vi "Main VI.vi"(8 "error in":errorcluster) -> (0 "error out":errorcluster)   [LabVIEW 2021]
doc: "Basic calculator built with LabVIEW"
uses:
  Controls/Queue Element.ctl
  Controls/Command Enum.ctl
  Controls/Storage Commands.ctl
  Controls/Storing Commands.ctl
  Controls/String Commands.ctl
  Controls/Operator String Control.ctl
  Controls/Operator Types.ctl
  Controls/String-Double Conversion Control.ctl
  Controls/Calculation Commands.ctl
panel:
  in  "Square":bool
  in  "Negate":bool
  in  "Clear All":bool
  in  "Clear Line":bool
  in  "Backspace":bool
  out "Secondary":string
  out "Primary":string
  in  "Square Root":bool
  in  "Reciprocal":bool
  in  "Equals":bool
  in  "Divide":bool
  in  "Multiply":bool
  in  "Subtract":bool
  in  "Add":bool
  in  "Decimal Point":bool
  in  "Button 0":bool
  in  "Button 9":bool
  in  "Button 8":bool
  in  "Button 7":bool
  in  "Button 6":bool
  in  "Button 5":bool
  in  "Button 4":bool
  in  "Button 3":bool
  in  "Button 2":bool
  in  "Button 1":bool
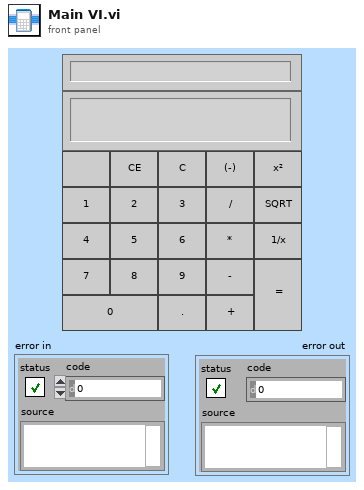
[diagram p1: front panel]
types:
  T1 = typedef "Queue Element.ctl" = cluster{"Command":T2, "Parameter":variant}
  T2 = typedef "Command Enum.ctl" = enum16{"Initialise", "Data Entry", "Decimal Point", "Operator", "Calculation", "Backspace", "Clear Line", "Clear All", "Close"}
  T3 = typedef "Operator String Control.ctl" = enum16{"GET", "Build", "Clear"}
  T4 = typedef "String Commands.ctl" = enum16{"GET Strings", "Set Secondary", "Build Primary", "Build Secondary", "Backspace", "Replace Operator", "Clear Primary", "Clear Secondary", "Clear ALL", "Decimal Point"}
  T5 = typedef "Storing Commands.ctl" = enum16{"Initialise", "GET", "SET"}
  T6 = typedef "Storage Commands.ctl" = enum16{"Initialise", "Build", "GET", "Reset"}
  T7 = typedef "Operator Types.ctl" = enum16{"Add", "Subtract", "Multiply", "Divide"}
  T8 = typedef "String-Double Conversion Control.ctl" = enum16{"String to DBL", "DBL to String"}
  T9 = typedef "Calculation Commands.ctl" = enum16{"Equals", "Square", "Square Root", "Reciprocal", "Negate"}
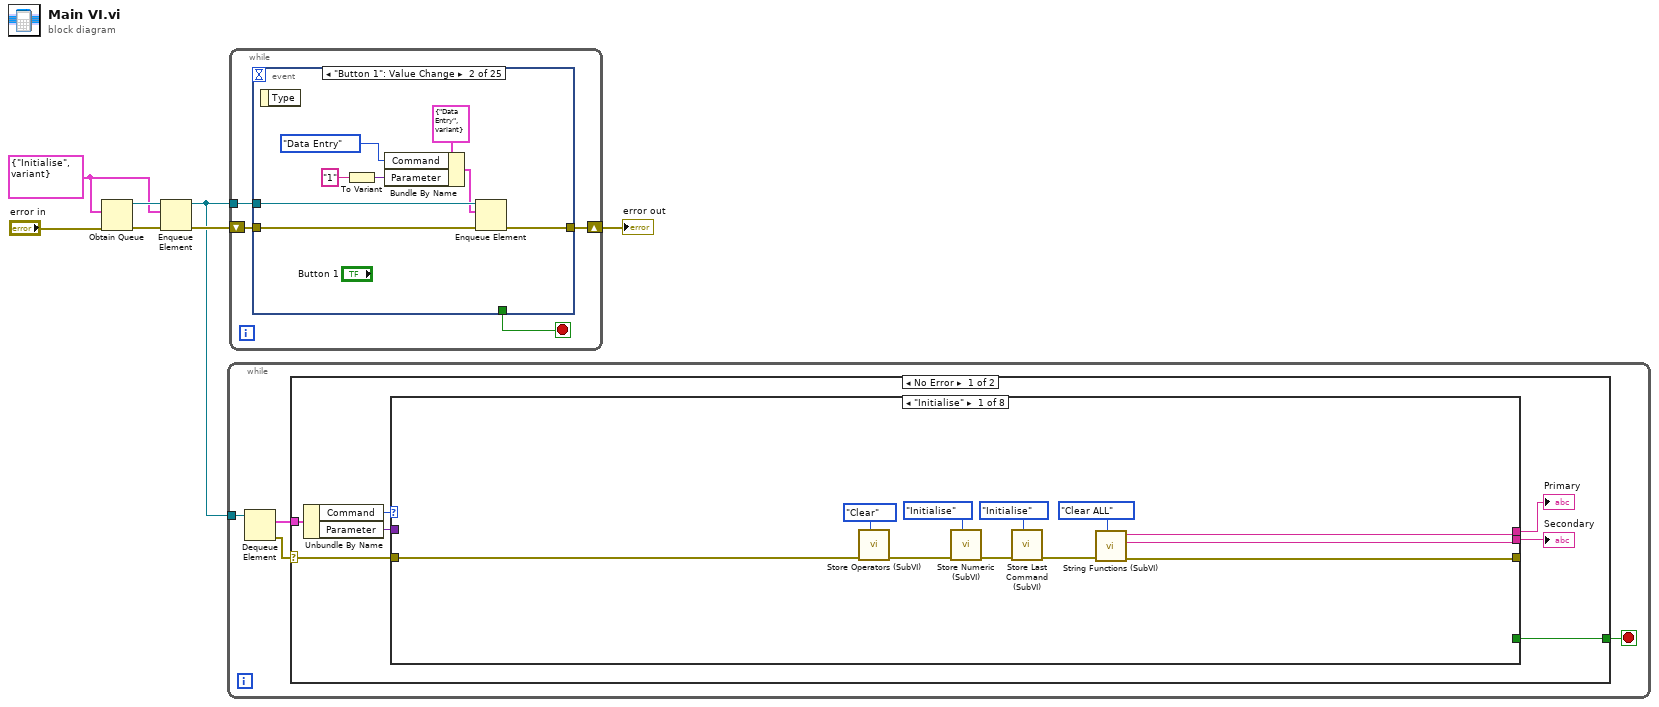
[diagram p0: block diagram]
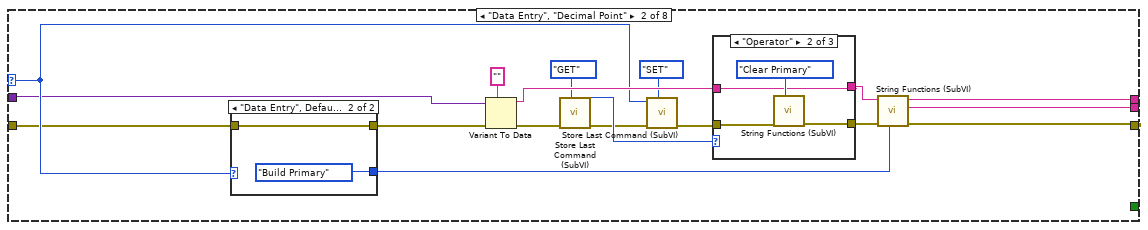
[diagram p2: hidden frame]
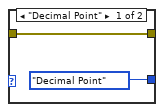
[diagram p3: hidden frame]
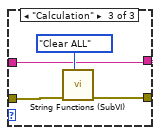
[diagram p5: hidden frame]
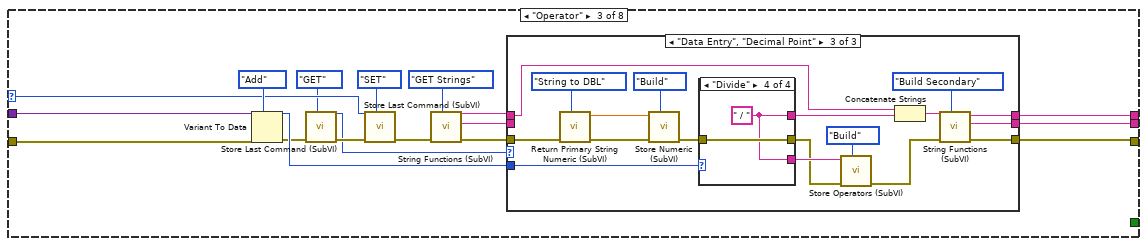
[diagram p6: hidden frame]
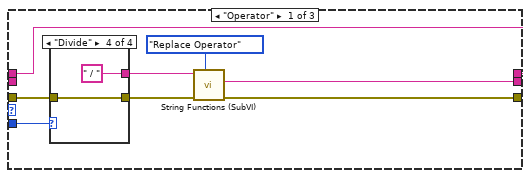
[diagram p7: hidden frame]
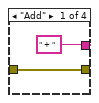
[diagram p8: hidden frame]
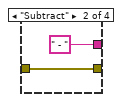
[diagram p9: hidden frame]
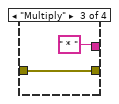
[diagram p10: hidden frame]
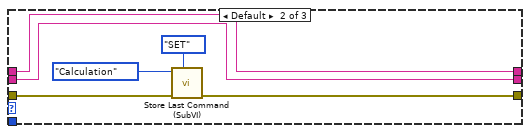
[diagram p11: hidden frame]
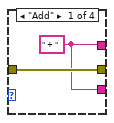
[diagram p12: hidden frame]
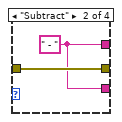
[diagram p13: hidden frame]
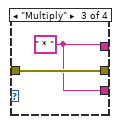
[diagram p14: hidden frame]
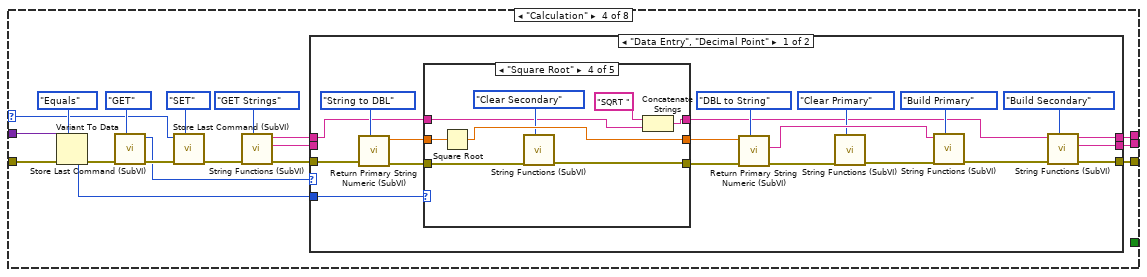
[diagram p15: hidden frame]
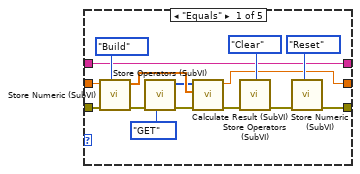
[diagram p16: hidden frame]
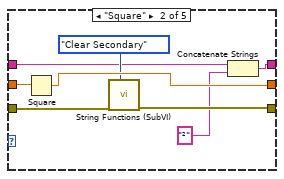
[diagram p17: hidden frame]
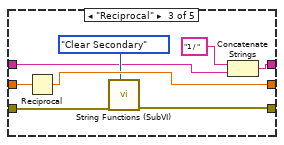
[diagram p18: hidden frame]
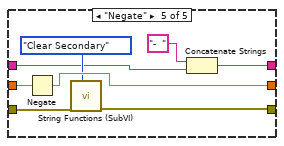
[diagram p19: hidden frame]
diagram:
  w6 = T1 {"Command"=enum."Initialise", "Parameter"=variant}
  n1 = Obtain Queue(element data type=w6, error in (no error)="error in") -> (queue out=w7:refnum<queue>, error out=w5:errorcluster)  [unwired: 3 in, 1 out]
  n2 = Enqueue Element(queue=w7, element=w6, error in (no error)=w5) -> (queue out=w2:refnum<queue>, error out=w4:errorcluster)  [unwired: 1 in, 1 out]
  n3 = while {
    tunnel: w2 -> [w11]
    stop <- w8 stop-if-true
    n4 = Dequeue Element(queue=w11) -> (element=w9:T1, error out=w10:errorcluster)  [unwired: 2 in, 2 out]
    n5 = case shown="No Error" w10 {
      selector: w10 -> [w12 _]
      tunnel: w9 -> [w18 _]
      tunnel: [w15 _] -> w8
      frame No Error {
        n6 = Unbundle By Name(w18) -> ("Command"=w17:T2, "Parameter"=w16:variant)
        n7 = case shown="\"Initialise\"" w17 {
          selector: w17 -> [_ w33 w72 w138 w217 w229 _ _]
          tunnel: w16 -> [_ w32 w78 w144 _ _ _ _]
          tunnel: [w19 w41 w75 w132 w223 w233 w241 w253] -> w14
          tunnel: [_ _ _ _ _ _ _ TRUE] -> w15
          tunnel: [w20 w42 w74 w131 w222 w232 w240 w252] -> w13
          tunnel: [w21 w34 w62 w128 w219 w227 w236 w255] -> _
          tunnel: w12 -> [w22 w31 w63 w127 w218 w228 w235 w254]
          frame "Initialise" {
            n8 = call "Store Operators (SubVI).vi"("Operator Command"=Operator_String_Control."Clear", "error in"=w22) -> ("error out"=w23:errorcluster)  [unwired: 8 in, 1 out]
            n9 = call "Store Numeric (SubVI).vi"("Commands"=Storage_Commands."Initialise", "error in"=w23) -> ("error out"=w27:errorcluster)  [unwired: 7 in, 2 out]
            n10 = call "Store Last Command (SubVI).vi"("Command"=Storing_Commands."Initialise", "error in"=w27) -> ("error out"=w26:errorcluster)  [unwired: 8 in, 1 out]
            n11 = call "String Functions (SubVI).vi"("String Function"=String_Commands."Clear ALL", "error in"=w26) -> ("error out"=w21:errorcluster, "Secondary Display String"=w20:string, "Primary Display String"=w19:string)  [unwired: 7 in]
          }
          frame "Data Entry", "Decimal Point" {
            n12 = case shown="\"Data Entry\", Default" w33 {
              tunnel: [String_Commands."Decimal Point" ("String Function") String_Commands."Build Primary" ("String Function")] -> w40
              tunnel: w31 -> [w48 w50]
              tunnel: [w48 w50] -> w30
              frame "Decimal Point" {
              }
              frame "Data Entry", Default {
              }
            }
            n13 = Variant To Data(error in=w30, type="", Variant=w32) -> (data=w46:string, error out=w44:errorcluster)
            n14 = call "Store Last Command (SubVI).vi"("Command"=Storing_Commands."GET", "error in"=w44) -> ("error out"=w36:errorcluster, "Last Command"=w43:T2)  [unwired: 8 in]
            n15 = call "Store Last Command (SubVI).vi"("Command"=Storing_Commands."SET", "error in"=w36, "Storage Command"=w33) -> ("error out"=w35:errorcluster)  [unwired: 7 in, 1 out]
            n16 = case shown="\"Operator\"" w43 {
              tunnel: w46 -> [w53 w54 w58]
              tunnel: w35 -> [w52 w56 w60]
              tunnel: [w52 w55 w59] -> w39
              tunnel: [w53 w54 w58] -> w38
              frame "Data Entry", Default {
              }
              frame "Operator" {
                n17 = call "String Functions (SubVI).vi"("String Function"=String_Commands."Clear Primary", "error in"=w56) -> ("error out"=w55:errorcluster)  [unwired: 7 in, 2 out]
              }
              frame "Calculation" {
                n18 = call "String Functions (SubVI).vi"("String Function"=String_Commands."Clear ALL", "error in"=w60) -> ("error out"=w59:errorcluster)  [unwired: 7 in, 2 out]
              }
            }
            n19 = call "String Functions (SubVI).vi"("String Function"=w40, "error in"=w39, "Function String"=w38) -> ("error out"=w34:errorcluster, "Secondary Display String"=w42:string, "Primary Display String"=w41:string)  [unwired: 6 in]
          }
          frame "Operator" {
            n20 = Variant To Data(error in=w63, type=Operator_Types."Add", Variant=w78) -> (data=w76:T7, error out=w71:errorcluster)
            n21 = call "Store Last Command (SubVI).vi"("Command"=Storing_Commands."GET") -> ("Last Command"=w69:T2)  [unwired: 9 in, 1 out]
            n22 = call "Store Last Command (SubVI).vi"("Command"=Storing_Commands."SET", "error in"=w71, "Storage Command"=w72) -> ("error out"=w68:errorcluster)  [unwired: 7 in, 1 out]
            n23 = call "String Functions (SubVI).vi"("String Function"=String_Commands."GET Strings", "error in"=w68) -> ("error out"=w64:errorcluster, "Secondary Display String"=w65:string, "Primary Display String"=w66:string)  [unwired: 7 in]
            n24 = case shown="\"Data Entry\", \"Decimal Point\"" w69 {
              tunnel: w76 -> [w83 _ w118]
              tunnel: [w86 w95 w116] -> w75
              tunnel: [w85 w96 w115] -> w74
              tunnel: w66 -> [w86 w95 w108]
              tunnel: w65 -> [_ w96 _]
              tunnel: w64 -> [w81 w100 w106]
              tunnel: [w79 w99 w107] -> w62
              frame "Operator" {
                n25 = case shown="\"Divide\"" w83 {
                  tunnel: [" + " ("New Char") " - " ("New Char") " * " ("New Char") " / " ("New Char")] -> w82
                  tunnel: w81 -> [w87 w89 w91 w93]
                  tunnel: [w87 w89 w91 w93] -> w80
                  frame "Add" {
                  }
                  frame "Subtract" {
                  }
                  frame "Multiply" {
                  }
                  frame "Divide" {
                  }
                }
                n26 = call "String Functions (SubVI).vi"("String Function"=String_Commands."Replace Operator", "error in"=w80, "Function String"=w82) -> ("error out"=w79:errorcluster, "Secondary Display String"=w85:string)  [unwired: 6 in, 1 out]
              }
              frame Default {
                n27 = call "Store Last Command (SubVI).vi"("Command"=Storing_Commands."SET", "error in"=w100, "Storage Command"=Command_Enum."Calculation") -> ("error out"=w99:errorcluster)  [unwired: 7 in, 1 out]
              }
              frame "Data Entry", "Decimal Point" {
                n28 = call "Return Primary String Numeric (SubVI).vi"("String-DBL Control"=String-Double_Conversion_Control."String to DBL", "error in"=w106) -> ("error out"=w114:errorcluster, "Primary Numeric"=w113:dbl)  [unwired: 7 in, 1 out]
                n29 = call "Store Numeric (SubVI).vi"("Commands"=Storage_Commands."Build", "error in"=w114, "Primary Numeric"=w113) -> ("error out"=w109:errorcluster)  [unwired: 6 in, 2 out]
                n30 = case shown="\"Divide\"" w118 {
                  tunnel: w109 -> [w120 w122 w124 w126]
                  tunnel: [w120 w122 w124 w126] -> w103
                  tunnel: [w119 w121 w123 w125] -> w110
                  tunnel: [w119 w121 w123 w125] -> w104
                  frame "Add" {
                    w119 = " + " ("New Char")
                  }
                  frame "Subtract" {
                    w121 = " - " ("New Char")
                  }
                  frame "Multiply" {
                    w123 = " * " ("New Char")
                  }
                  frame "Divide" {
                    w125 = " / " ("New Char")
                  }
                }
                n31 = call "Store Operators (SubVI).vi"("Operator Command"=Operator_String_Control."Build", "error in"=w103, "Operator"=w104) -> ("error out"=w102:errorcluster)  [unwired: 7 in, 1 out]
                n32 = Concatenate Strings(w108, w110) -> (w111:string)
                n33 = call "String Functions (SubVI).vi"("String Function"=String_Commands."Build Secondary", "error in"=w102, "Function String"=w111) -> ("error out"=w107:errorcluster, "Secondary Display String"=w115:string, "Primary Display String"=w116:string)  [unwired: 6 in]
              }
            }
          }
          frame "Calculation" {
            n34 = Variant To Data(error in=w127, type=Calculation_Commands."Equals", Variant=w144) -> (data=w136:T9, error out=w140:errorcluster)
            n35 = call "Store Last Command (SubVI).vi"("Command"=Storing_Commands."GET", "error in"=w140) -> ("error out"=w139:errorcluster, "Last Command"=w137:T2)  [unwired: 8 in]
            n36 = call "Store Last Command (SubVI).vi"("Command"=Storing_Commands."SET", "error in"=w139, "Storage Command"=w138) -> ("error out"=w135:errorcluster)  [unwired: 7 in, 1 out]
            n37 = call "String Functions (SubVI).vi"("String Function"=String_Commands."GET Strings", "error in"=w135) -> ("error out"=w129:errorcluster, "Secondary Display String"=w130:string, "Primary Display String"=w133:string)  [unwired: 7 in]
            n38 = case shown="\"Data Entry\", \"Decimal Point\"" w137 {
              tunnel: w136 -> [w164 _]
              tunnel: w133 -> [w146 w213]
              tunnel: [w162 w213] -> w132
              tunnel: [w161 w214] -> w131
              tunnel: w130 -> [_ w214]
              tunnel: w129 -> [w157 w212]
              tunnel: [w160 w212] -> w128
              frame "Data Entry", "Decimal Point" {
                n39 = call "Return Primary String Numeric (SubVI).vi"("String-DBL Control"=String-Double_Conversion_Control."String to DBL", "error in"=w157) -> ("error out"=w156:errorcluster, "Primary Numeric"=w159:dbl)  [unwired: 7 in, 1 out]
                n40 = case shown="\"Square Root\"" w164 {
                  tunnel: [w168 w184 w192 w200 w208] -> w148
                  tunnel: w156 -> [w179 w185 w193 w201 w209]
                  tunnel: w159 -> [w177 w187 w195 w203 w211]
                  tunnel: [w166 w186 w194 w202 w210] -> w149
                  tunnel: w146 -> [w165 w182 w189 w197 w205]
                  tunnel: [w165 w181 w190 w198 w206] -> w145
                  frame "Equals" {
                    n41 = call "Store Numeric (SubVI).vi"("Commands"=Storage_Commands."Build", "error in"=w179, "Primary Numeric"=w177) -> ("error out"=w176:errorcluster, "Stored Values"=w174:dbl[])  [unwired: 6 in, 1 out]
                    n42 = call "Store Operators (SubVI).vi"("Operator Command"=Operator_String_Control."GET", "error in"=w176) -> ("error out"=w173:errorcluster, "Operator Array"=w172:T7[])  [unwired: 8 in]
                    n43 = call "Calculate Result (SubVI).vi"("error in"=w173, "Stored Values"=w174, "Operator Array"=w172) -> ("error out"=w171:errorcluster, "Result"=w166:dbl)  [unwired: 7 in]
                    n44 = call "Store Operators (SubVI).vi"("Operator Command"=Operator_String_Control."Clear", "error in"=w171) -> ("error out"=w169:errorcluster)  [unwired: 8 in, 1 out]
                    n45 = call "Store Numeric (SubVI).vi"("Commands"=Storage_Commands."Reset", "error in"=w169) -> ("error out"=w168:errorcluster)  [unwired: 7 in, 2 out]
                  }
                  frame "Square" {
                    n46 = Square(x=w187) -> (x^2=w186:dbl)
                    n47 = call "String Functions (SubVI).vi"("String Function"=String_Commands."Clear Secondary", "error in"=w185) -> ("error out"=w184:errorcluster)  [unwired: 7 in, 2 out]
                    n48 = Concatenate Strings(w182, "²") -> (w181:string)
                  }
                  frame "Reciprocal" {
                    n49 = Reciprocal(x=w195) -> (1/x=w194:dbl)
                    n50 = call "String Functions (SubVI).vi"("String Function"=String_Commands."Clear Secondary", "error in"=w193) -> ("error out"=w192:errorcluster)  [unwired: 7 in, 2 out]
                    n51 = Concatenate Strings("1 / ", w189) -> (w190:string)
                  }
                  frame "Square Root" {
                    n52 = Square Root(x=w203) -> (sqrt(x)=w202:dbl)
                    n53 = call "String Functions (SubVI).vi"("String Function"=String_Commands."Clear Secondary", "error in"=w201) -> ("error out"=w200:errorcluster)  [unwired: 7 in, 2 out]
                    n54 = Concatenate Strings("SQRT ", w197) -> (w198:string)
                  }
                  frame "Negate" {
                    n55 = Negate(x=w211) -> (-x=w210:dbl)
                    n56 = call "String Functions (SubVI).vi"("String Function"=String_Commands."Clear Secondary", "error in"=w209) -> ("error out"=w208:errorcluster)  [unwired: 7 in, 2 out]
                    n57 = Concatenate Strings("-  ", w205) -> (w206:string)
                  }
                }
                n58 = call "Return Primary String Numeric (SubVI).vi"("String-DBL Control"=String-Double_Conversion_Control."DBL to String", "error in"=w148, "Primary Numeric"=w149) -> ("error out"=w153:errorcluster, "Primary String"=w155:string)  [unwired: 6 in, 1 out]
                n59 = call "String Functions (SubVI).vi"("String Function"=String_Commands."Clear Primary", "error in"=w153) -> ("error out"=w154:errorcluster)  [unwired: 7 in, 2 out]
                n60 = call "String Functions (SubVI).vi"("String Function"=String_Commands."Build Primary", "error in"=w154, "Function String"=w155) -> ("error out"=w147:errorcluster)  [unwired: 6 in, 2 out]
                n61 = call "String Functions (SubVI).vi"("String Function"=String_Commands."Build Secondary", "error in"=w147, "Function String"=w145) -> ("error out"=w160:errorcluster, "Secondary Display String"=w161:string, "Primary Display String"=w162:string)  [unwired: 6 in]
              }
              frame Default {
              }
            }
          }
          frame "Clear Line" {
            n62 = call "Store Last Command (SubVI).vi"("Command"=Storing_Commands."GET") -> ("Last Command"=w215:T2)  [unwired: 9 in, 1 out]
            n63 = call "Store Last Command (SubVI).vi"("Command"=Storing_Commands."SET", "error in"=w218, "Storage Command"=w217) -> ("error out"=w220:errorcluster)  [unwired: 7 in, 1 out]
            n64 = case shown="\"Calculation\"" w215 {
              tunnel: [String_Commands."Clear ALL" ("String Function") String_Commands."Clear Primary" ("String Function")] -> w224
              frame "Calculation" {
              }
              frame Default {
              }
            }
            n65 = call "String Functions (SubVI).vi"("String Function"=w224, "error in"=w220) -> ("error out"=w219:errorcluster, "Secondary Display String"=w222:string, "Primary Display String"=w223:string)  [unwired: 7 in]
          }
          frame "Clear All" {
            n66 = call "Store Last Command (SubVI).vi"("Command"=Storing_Commands."SET", "error in"=w228, "Storage Command"=w229) -> ("error out"=w231:errorcluster)  [unwired: 7 in, 1 out]
            n67 = call "String Functions (SubVI).vi"("String Function"=String_Commands."Clear ALL", "error in"=w231) -> ("error out"=w227:errorcluster, "Secondary Display String"=w232:string, "Primary Display String"=w233:string)  [unwired: 7 in]
          }
          frame "Backspace" {
            n68 = call "Store Last Command (SubVI).vi"("Command"=Storing_Commands."GET", "error in"=w235) -> ("error out"=w239:errorcluster, "Last Command"=w237:T2)  [unwired: 8 in]
            n69 = case shown="\"Data Entry\", \"Decimal Point\"" w237 {
              tunnel: w239 -> [w246 w250]
              tunnel: [w244 w249] -> w241
              tunnel: [w243 w248] -> w240
              tunnel: [w242 w247] -> w236
              frame Default {
                n70 = call "String Functions (SubVI).vi"("String Function"=String_Commands."GET Strings", "error in"=w246) -> ("error out"=w242:errorcluster, "Secondary Display String"=w243:string, "Primary Display String"=w244:string)  [unwired: 7 in]
              }
              frame "Data Entry", "Decimal Point" {
                n71 = call "String Functions (SubVI).vi"("String Function"=String_Commands."Backspace", "error in"=w250) -> ("error out"=w247:errorcluster, "Secondary Display String"=w248:string, "Primary Display String"=w249:string)  [unwired: 7 in]
              }
            }
          }
          frame "Close" {
            n72 = call "Store Operators (SubVI).vi"("Operator Command"=Operator_String_Control."Clear", "error in"=w254) -> ("error out"=w256:errorcluster)  [unwired: 8 in, 1 out]
            n73 = call "Store Numeric (SubVI).vi"("Commands"=Storage_Commands."Initialise", "error in"=w256) -> ("error out"=w260:errorcluster)  [unwired: 7 in, 2 out]
            n74 = call "Store Last Command (SubVI).vi"("Command"=Storing_Commands."Initialise", "error in"=w260) -> ("error out"=w259:errorcluster)  [unwired: 8 in, 1 out]
            n75 = call "String Functions (SubVI).vi"("String Function"=String_Commands."Clear ALL", "error in"=w259) -> ("error out"=w255:errorcluster, "Secondary Display String"=w252:string, "Primary Display String"=w253:string)  [unwired: 7 in]
          }
        }
        "Primary" <- w14
        "Secondary" <- w13
      }
      frame Error {
      }
    }
  }
  n76 = while {
    tunnel: w2 -> [w267]
    shift-right: [w265] -> w3
    shift-left: w4 -> [w266]
    stop <- w264 stop-if-true
    n77 = event shown="[1] \"Button 1\": Value Change" {
      selector: _ -> [_ _ _ _ _ _ _ _ _ _ _ _ _ _ _ _ _ _ _ _ _ _ _ _ _]
      dyn-events: _ -> [_ _ _ _ _ _ _ _ _ _ _ _ _ _ _ _ _ _ _ _ _ _ _ _ _]
      timeout: _ -> [_ _ _ _ _ _ _ _ _ _ _ _ _ _ _ _ _ _ _ _ _ _ _ _ _]
      tunnel: w267 -> [_ w276 w284 w292 w300 w308 w316 w324 w332 w340 w348 w356 w364 w372 w380 w388 w394 w400 w406 w414 w422 w430 w438 w446 w448]
      tunnel: w266 -> [w268 w271 w279 w287 w295 w303 w311 w319 w327 w335 w343 w351 w360 w368 w376 w384 w391 w397 w403 w411 w419 w427 w435 w443 w451]
      tunnel: [w268 w270 w278 w286 w294 w302 w310 w318 w326 w334 w342 w350 w359 w367 w375 w383 w390 w396 w402 w410 w418 w426 w434 w442 w449] -> w265
      tunnel: [_ _ _ _ _ _ _ _ _ _ _ _ _ _ _ _ _ _ _ _ _ _ _ _ w450] -> w264
      event Timeout {
        n78 = event-data() -> ()  [unwired: 1 in, 1 out]
      }
      event "Button 1": Value Change {
        n79 = event-data() -> ()  [unwired: 1 in, 1 out]
        n80 = To Variant(anything="1") -> (Variant=w273:variant)
        n81 = Bundle By Name(cluster=T1 {"Command"=enum."Data Entry", "Parameter"=variant}, "Command"=Command_Enum."Data Entry", "Parameter"=w273) -> (w272:T1)
        n82 = Enqueue Element(queue=w276, element=w272, error in (no error)=w271) -> (error out=w270:errorcluster)  [unwired: 1 in, 2 out]
      }
      event "Button 2": Value Change {
        n83 = event-data() -> ()  [unwired: 1 in, 1 out]
        n84 = To Variant(anything="2") -> (Variant=w281:variant)
        n85 = Bundle By Name(cluster=T1 {"Command"=enum."Data Entry", "Parameter"=variant}, "Command"=Command_Enum."Data Entry", "Parameter"=w281) -> (w280:T1)
        n86 = Enqueue Element(queue=w284, element=w280, error in (no error)=w279) -> (error out=w278:errorcluster)  [unwired: 1 in, 2 out]
      }
      event "Button 3": Value Change {
        n87 = event-data() -> ()  [unwired: 1 in, 1 out]
        n88 = To Variant(anything="3") -> (Variant=w289:variant)
        n89 = Bundle By Name(cluster=T1 {"Command"=enum."Data Entry", "Parameter"=variant}, "Command"=Command_Enum."Data Entry", "Parameter"=w289) -> (w288:T1)
        n90 = Enqueue Element(queue=w292, element=w288, error in (no error)=w287) -> (error out=w286:errorcluster)  [unwired: 1 in, 2 out]
      }
      event "Button 4": Value Change {
        n91 = event-data() -> ()  [unwired: 1 in, 1 out]
        n92 = To Variant(anything="4") -> (Variant=w297:variant)
        n93 = Bundle By Name(cluster=T1 {"Command"=enum."Data Entry", "Parameter"=variant}, "Command"=Command_Enum."Data Entry", "Parameter"=w297) -> (w296:T1)
        n94 = Enqueue Element(queue=w300, element=w296, error in (no error)=w295) -> (error out=w294:errorcluster)  [unwired: 1 in, 2 out]
      }
      event "Button 5": Value Change {
        n95 = event-data() -> ()  [unwired: 1 in, 1 out]
        n96 = To Variant(anything="5") -> (Variant=w305:variant)
        n97 = Bundle By Name(cluster=T1 {"Command"=enum."Data Entry", "Parameter"=variant}, "Command"=Command_Enum."Data Entry", "Parameter"=w305) -> (w304:T1)
        n98 = Enqueue Element(queue=w308, element=w304, error in (no error)=w303) -> (error out=w302:errorcluster)  [unwired: 1 in, 2 out]
      }
      event "Button 6": Value Change {
        n99 = event-data() -> ()  [unwired: 1 in, 1 out]
        n100 = To Variant(anything="6") -> (Variant=w313:variant)
        n101 = Bundle By Name(cluster=T1 {"Command"=enum."Data Entry", "Parameter"=variant}, "Command"=Command_Enum."Data Entry", "Parameter"=w313) -> (w312:T1)
        n102 = Enqueue Element(queue=w316, element=w312, error in (no error)=w311) -> (error out=w310:errorcluster)  [unwired: 1 in, 2 out]
      }
      event "Button 7": Value Change {
        n103 = event-data() -> ()  [unwired: 1 in, 1 out]
        n104 = To Variant(anything="7") -> (Variant=w321:variant)
        n105 = Bundle By Name(cluster=T1 {"Command"=enum."Data Entry", "Parameter"=variant}, "Command"=Command_Enum."Data Entry", "Parameter"=w321) -> (w320:T1)
        n106 = Enqueue Element(queue=w324, element=w320, error in (no error)=w319) -> (error out=w318:errorcluster)  [unwired: 1 in, 2 out]
      }
      event "Button 8": Value Change {
        n107 = event-data() -> ()  [unwired: 1 in, 1 out]
        n108 = To Variant(anything="8") -> (Variant=w329:variant)
        n109 = Bundle By Name(cluster=T1 {"Command"=enum."Data Entry", "Parameter"=variant}, "Command"=Command_Enum."Data Entry", "Parameter"=w329) -> (w328:T1)
        n110 = Enqueue Element(queue=w332, element=w328, error in (no error)=w327) -> (error out=w326:errorcluster)  [unwired: 1 in, 2 out]
      }
      event "Button 9": Value Change {
        n111 = event-data() -> ()  [unwired: 1 in, 1 out]
        n112 = To Variant(anything="9") -> (Variant=w337:variant)
        n113 = Bundle By Name(cluster=T1 {"Command"=enum."Data Entry", "Parameter"=variant}, "Command"=Command_Enum."Data Entry", "Parameter"=w337) -> (w336:T1)
        n114 = Enqueue Element(queue=w340, element=w336, error in (no error)=w335) -> (error out=w334:errorcluster)  [unwired: 1 in, 2 out]
      }
      event "Button 0": Value Change {
        n115 = event-data() -> ()  [unwired: 1 in, 1 out]
        n116 = To Variant(anything="0") -> (Variant=w345:variant)
        n117 = Bundle By Name(cluster=T1 {"Command"=enum."Data Entry", "Parameter"=variant}, "Command"=Command_Enum."Data Entry", "Parameter"=w345) -> (w344:T1)
        n118 = Enqueue Element(queue=w348, element=w344, error in (no error)=w343) -> (error out=w342:errorcluster)  [unwired: 1 in, 2 out]
      }
      event "Decimal Point": Value Change {
        n119 = event-data() -> ()  [unwired: 1 in, 1 out]
        n120 = To Variant(anything=".") -> (Variant=w353:variant)
        n121 = Bundle By Name(cluster=T1 {"Command"=enum."Data Entry", "Parameter"=variant}, "Command"=Command_Enum."Decimal Point", "Parameter"=w353) -> (w352:T1)
        n122 = Enqueue Element(queue=w356, element=w352, error in (no error)=w351) -> (error out=w350:errorcluster)  [unwired: 1 in, 2 out]
      }
      event "Add": Value Change {
        n123 = event-data() -> ()  [unwired: 1 in, 1 out]
        n124 = To Variant(anything=Operator_Types."Add") -> (Variant=w362:variant)
        n125 = Bundle By Name(cluster=T1 {"Command"=enum."Data Entry", "Parameter"=variant}, "Command"=Command_Enum."Operator", "Parameter"=w362) -> (w361:T1)
        n126 = Enqueue Element(queue=w364, element=w361, error in (no error)=w360) -> (error out=w359:errorcluster)  [unwired: 1 in, 2 out]
      }
      event "Subtract": Value Change {
        n127 = event-data() -> ()  [unwired: 1 in, 1 out]
        n128 = To Variant(anything=Operator_Types."Subtract") -> (Variant=w370:variant)
        n129 = Bundle By Name(cluster=T1 {"Command"=enum."Data Entry", "Parameter"=variant}, "Command"=Command_Enum."Operator", "Parameter"=w370) -> (w369:T1)
        n130 = Enqueue Element(queue=w372, element=w369, error in (no error)=w368) -> (error out=w367:errorcluster)  [unwired: 1 in, 2 out]
      }
      event "Multiply": Value Change {
        n131 = event-data() -> ()  [unwired: 1 in, 1 out]
        n132 = To Variant(anything=Operator_Types."Multiply") -> (Variant=w378:variant)
        n133 = Bundle By Name(cluster=T1 {"Command"=enum."Data Entry", "Parameter"=variant}, "Command"=Command_Enum."Operator", "Parameter"=w378) -> (w377:T1)
        n134 = Enqueue Element(queue=w380, element=w377, error in (no error)=w376) -> (error out=w375:errorcluster)  [unwired: 1 in, 2 out]
      }
      event "Divide": Value Change {
        n135 = event-data() -> ()  [unwired: 1 in, 1 out]
        n136 = To Variant(anything=Operator_Types."Divide") -> (Variant=w386:variant)
        n137 = Bundle By Name(cluster=T1 {"Command"=enum."Data Entry", "Parameter"=variant}, "Command"=Command_Enum."Operator", "Parameter"=w386) -> (w385:T1)
        n138 = Enqueue Element(queue=w388, element=w385, error in (no error)=w384) -> (error out=w383:errorcluster)  [unwired: 1 in, 2 out]
      }
      event "Clear All": Value Change {
        n139 = event-data() -> ()  [unwired: 1 in, 1 out]
        n140 = Bundle By Name(cluster=T1 {"Command"=enum."Data Entry", "Parameter"=variant}, "Command"=Command_Enum."Clear All") -> (w392:T1)
        n141 = Enqueue Element(queue=w394, element=w392, error in (no error)=w391) -> (error out=w390:errorcluster)  [unwired: 1 in, 2 out]
      }
      event "Clear Line": Value Change {
        n142 = event-data() -> ()  [unwired: 1 in, 1 out]
        n143 = Bundle By Name(cluster=T1 {"Command"=enum."Data Entry", "Parameter"=variant}, "Command"=Command_Enum."Clear Line") -> (w398:T1)
        n144 = Enqueue Element(queue=w400, element=w398, error in (no error)=w397) -> (error out=w396:errorcluster)  [unwired: 1 in, 2 out]
      }
      event "Backspace": Value Change {
        n145 = event-data() -> ()  [unwired: 1 in, 1 out]
        n146 = Bundle By Name(cluster=T1 {"Command"=enum."Data Entry", "Parameter"=variant}, "Command"=Command_Enum."Backspace") -> (w404:T1)
        n147 = Enqueue Element(queue=w406, element=w404, error in (no error)=w403) -> (error out=w402:errorcluster)  [unwired: 1 in, 2 out]
      }
      event "Equals": Value Change {
        n148 = event-data() -> ()  [unwired: 1 in, 1 out]
        n149 = To Variant(anything=Calculation_Commands."Equals") -> (Variant=w408:variant)
        n150 = Bundle By Name(cluster=T1 {"Command"=enum."Data Entry", "Parameter"=variant}, "Command"=Command_Enum."Calculation", "Parameter"=w408) -> (w412:T1)
        n151 = Enqueue Element(queue=w414, element=w412, error in (no error)=w411) -> (error out=w410:errorcluster)  [unwired: 1 in, 2 out]
      }
      event "Square Root": Value Change {
        n152 = event-data() -> ()  [unwired: 1 in, 1 out]
        n153 = To Variant(anything=Calculation_Commands."Square Root") -> (Variant=w416:variant)
        n154 = Bundle By Name(cluster=T1 {"Command"=enum."Data Entry", "Parameter"=variant}, "Command"=Command_Enum."Calculation", "Parameter"=w416) -> (w420:T1)
        n155 = Enqueue Element(queue=w422, element=w420, error in (no error)=w419) -> (error out=w418:errorcluster)  [unwired: 1 in, 2 out]
      }
      event "Reciprocal": Value Change {
        n156 = event-data() -> ()  [unwired: 1 in, 1 out]
        n157 = To Variant(anything=Calculation_Commands."Reciprocal") -> (Variant=w424:variant)
        n158 = Bundle By Name(cluster=T1 {"Command"=enum."Data Entry", "Parameter"=variant}, "Command"=Command_Enum."Calculation", "Parameter"=w424) -> (w428:T1)
        n159 = Enqueue Element(queue=w430, element=w428, error in (no error)=w427) -> (error out=w426:errorcluster)  [unwired: 1 in, 2 out]
      }
      event "Square": Value Change {
        n160 = event-data() -> ()  [unwired: 1 in, 1 out]
        n161 = To Variant(anything=Calculation_Commands."Square") -> (Variant=w432:variant)
        n162 = Bundle By Name(cluster=T1 {"Command"=enum."Data Entry", "Parameter"=variant}, "Command"=Command_Enum."Calculation", "Parameter"=w432) -> (w436:T1)
        n163 = Enqueue Element(queue=w438, element=w436, error in (no error)=w435) -> (error out=w434:errorcluster)  [unwired: 1 in, 2 out]
      }
      event "Negate": Value Change {
        n164 = event-data() -> ()  [unwired: 1 in, 1 out]
        n165 = To Variant(anything=Calculation_Commands."Negate") -> (Variant=w440:variant)
        n166 = Bundle By Name(cluster=T1 {"Command"=enum."Data Entry", "Parameter"=variant}, "Command"=Command_Enum."Calculation", "Parameter"=w440) -> (w444:T1)
        n167 = Enqueue Element(queue=w446, element=w444, error in (no error)=w443) -> (error out=w442:errorcluster)  [unwired: 1 in, 2 out]
      }
      event Panel Close? {
        w450 = TRUE
        n168 = event-data() -> ()  [unwired: 1 in, 1 out]
        n169 = Enqueue Element(queue=w448, element=T1 {"Command"=enum."Close", "Parameter"=variant}, error in (no error)=w451) -> (error out=w449:errorcluster)  [unwired: 1 in, 2 out]
        n170 = event-data("Discard?"=w450) -> ()  [unwired: 1 in, 1 out]
      }
    }
  }
  "error out" <- w3
